vi "Multicore Simulator.vi"() -> ()   [LabVIEW 2016]
uses:
  Z:/LiSARD_Reference_Project/Multicore_1.6beta/CodeConverter/Controls/CommandLine.ctl
  Z:/LiSARD_Reference_Project/Multicore_1.6beta/CodeConverter/Controls/EX.Command.ctl
  Z:/LiSARD_Reference_Project/Multicore_1.6beta/CodeConverter/Controls/WB.Operation.ctl
  Z:/LiSARD_Reference_Project/Multicore_1.6beta/CodeConverter/SoftCoreCodeConverter.lvlib
panel:
  out "Output":dbl[](array[numeric])=[0.0, 1.0, 2.0, 3.0, 4.0, 5.0, 6.0, 7.0, 8.0, 9.0, 10.0, 11.0, 12.0, 13.0, 14.0, 15.0, 16.0, 17.0, 18.0, 19.0, 20.0, 21.0, 22.0, 23.0, 24.0, 25.0, 26.0, 27.0, 28.0, 29.0, 30.0, 0.0, 0.0, 0.0, 0.0, 0.0, 0.0, 0.0, 0.0, 0.0, 0.0, 0.0, 0.0, 0.0, 0.0, 0.0, 0.0, 0.0, 0.0, 0.0, 0.0, 0.0, 0.0, 0.0, 0.0, 0.0, 0.0, 0.0, 0.0, 0.0, 0.0, 0.0, 0.0, 0.0, 0.0, 0.0, 0.0, 0.0, 0.0, 0.0, 0.0, 0.0, 0.0, 0.0, 0.0, 0.0, 0.0, 0.0, 0.0, 0.0, 0.0, 0.0, 0.0, 0.0, 0.0, 0.0, 0.0, 0.0, 0.0, 0.0, 0.0, 0.0, 0.0, 0.0, 0.0, 0.0, 0.0, 0.0, 0.0, 0.0, 0.0, 0.0, 0.0, 0.0, 0.0, 0.0, 0.0, 0.0, 0.0, 0.0, 0.0, 0.0, 0.0, 0.0, 0.0, 0.0, 0.0, 0.0, 0.0, 0.0, 0.0, 0.0, 0.0, 0.0, 0.0, 0.0, 0.0, 0.0, 0.0, 0.0, 0.0, 0.0, 0.0, 0.0, 0.0, 0.0, 0.0, 0.0, 0.0, 0.0, 0.0, 0.0, 0.0, 0.0, 0.0, 0.0, 0.0, 0.0, 0.0, 0.0, 0.0, 0.0, 0.0, 0.0, 0.0, 0.0, 0.0, 0.0, 0.0, 0.0, 0.0, 0.0, 0.0, 0.0, 0.0, 0.0, 0.0, 0.0, 0.0, 0.0, 0.0, 0.0, 0.0, 0.0, 0.0, 0.0, 0.0, 0.0, 0.0, 0.0, 0.0, 0.0, 0.0, 0.0, 0.0, 0.0, 0.0, 0.0, 0.0, 0.0, 0.0, 0.0, 0.0, 0.0, 0.0, 0.0, 0.0, 0.0, 0.0, 0.0, 0.0, 0.0, 0.0, 0.0, 0.0, 0.0, 0.0, 0.0, 0.0, 0.0, 0.0, 0.0, 0.0, 0.0, 0.0, 0.0, 0.0, 0.0, 0.0, 0.0, 0.0, 0.0, 0.0, 0.0, 0.0, 0.0, 0.0, 0.0, 0.0, 0.0, 0.0, 0.0, 0.0, 0.0, 0.0, 0.0, 0.0, 0.0, 0.0, 0.0, 0.0, 0.0, 0.0, 0.0, 0.0, 0.0, 0.0, 0.0, 0.0, 0.0, 0.0, 0.0, 0.0, 0.0, 0.0]
  in  "CoreCode":T1[][](array[typedef])=[[{"Ex.Command"=enum."None", "Ex.AddressIn1"=1.0, "Ex.AddressIn2"=2.0, "WB.Command"=enum."Add", "WB.AddressOut"=3.0, "Bypass1"=0.0, "Bypass 2"=0.0}, {"Ex.Command"=enum."None", "Ex.AddressIn1"=9.0, "Ex.AddressIn2"=10.0, "WB.Command"=enum."Add", "WB.AddressOut"=11.0, "Bypass1"=0.0, "Bypass 2"=0.0}, {"Ex.Command"=enum."None", "Ex.AddressIn1"=23.0, "Ex.AddressIn2"=17.0, "WB.Command"=enum."Mul", "WB.AddressOut"=18.0, "Bypass1"=0.0, "Bypass 2"=0.0}, {"Ex.Command"=enum."None", "Ex.AddressIn1"=23.0, "Ex.AddressIn2"=23.0, "WB.Command"=enum."Mul", "WB.AddressOut"=24.0, "Bypass1"=0.0, "Bypass 2"=0.0}], [{"Ex.Command"=enum."None", "Ex.AddressIn1"=4.0, "Ex.AddressIn2"=5.0, "WB.Command"=enum."Mul", "WB.AddressOut"=6.0, "Bypass1"=0.0, "Bypass 2"=0.0}, {"Ex.Command"=enum."None", "Ex.AddressIn1"=11.0, "Ex.AddressIn2"=11.0, "WB.Command"=enum."Mul", "WB.AddressOut"=12.0, "Bypass1"=0.0, "Bypass 2"=0.0}, {"Ex.Command"=enum."None", "Ex.AddressIn1"=18.0, "Ex.AddressIn2"=18.0, "WB.Command"=enum."Mul", "WB.AddressOut"=19.0, "Bypass1"=0.0, "Bypass 2"=0.0}, {"Ex.Command"=enum."None", "Ex.AddressIn1"=23.0, "Ex.AddressIn2"=25.0, "WB.Command"=enum."Mul", "WB.AddressOut"=26.0, "Bypass1"=0.0, "Bypass 2"=0.0}], [{"Ex.Command"=enum."None", "Ex.AddressIn1"=3.0, "Ex.AddressIn2"=6.0, "WB.Command"=enum."Add", "WB.AddressOut"=7.0, "Bypass1"=0.0, "Bypass 2"=0.0}, {"Ex.Command"=enum."Sub", "Ex.AddressIn1"=13.0, "Ex.AddressIn2"=14.0, "WB.Command"=enum."Sub", "WB.AddressOut"=15.0, "Bypass1"=0.0, "Bypass 2"=0.0}, {"Ex.Command"=enum."None", "Ex.AddressIn1"=24.0, "Ex.AddressIn2"=20.0, "WB.Command"=enum."Add", "WB.AddressOut"=20.0, "Bypass1"=0.0, "Bypass 2"=0.0}, {"Ex.Command"=enum."Sub", "Ex.AddressIn1"=24.0, "Ex.AddressIn2"=26.0, "WB.Command"=enum."Sub", "WB.AddressOut"=27.0, "Bypass1"=0.0, "Bypass 2"=0.0}], [{"Ex.Command"=enum."None", "Ex.AddressIn1"=7.0, "Ex.AddressIn2"=8.0, "WB.Command"=enum."Mov", "WB.AddressOut"=1.0, "Bypass1"=3.0, "Bypass 2"=0.0}, {"Ex.Command"=enum."None", "Ex.AddressIn1"=15.0, "Ex.AddressIn2"=15.0, "WB.Command"=enum."Mul", "WB.AddressOut"=16.0, "Bypass1"=0.0, "Bypass 2"=0.0}, {"Ex.Command"=enum."None", "Ex.AddressIn1"=19.0, "Ex.AddressIn2"=20.0, "WB.Command"=enum."Add", "WB.AddressOut"=22.0, "Bypass1"=0.0, "Bypass 2"=0.0}, {"Ex.Command"=enum."None", "Ex.AddressIn1"=25.0, "Ex.AddressIn2"=25.0, "WB.Command"=enum."Mul", "WB.AddressOut"=28.0, "Bypass1"=0.0, "Bypass 2"=0.0}], [{"Ex.Command"=enum."Sub", "Ex.AddressIn1"=1.0, "Ex.AddressIn2"=4.0, "WB.Command"=enum."Sub", "WB.AddressOut"=2.0, "Bypass1"=0.0, "Bypass 2"=0.0}, {"Ex.Command"=enum."Sub", "Ex.AddressIn1"=12.0, "Ex.AddressIn2"=16.0, "WB.Command"=enum."Sub", "WB.AddressOut"=10.0, "Bypass1"=0.0, "Bypass 2"=0.0}, {"Ex.Command"=enum."None", "Ex.AddressIn1"=22.0, "Ex.AddressIn2"=23.0, "WB.Command"=enum."Mov", "WB.AddressOut"=21.0, "Bypass1"=0.0, "Bypass 2"=0.0}, {"Ex.Command"=enum."None", "Ex.AddressIn1"=27.0, "Ex.AddressIn2"=28.0, "WB.Command"=enum."Add", "WB.AddressOut"=29.0, "Bypass1"=0.0, "Bypass 2"=0.0}]]
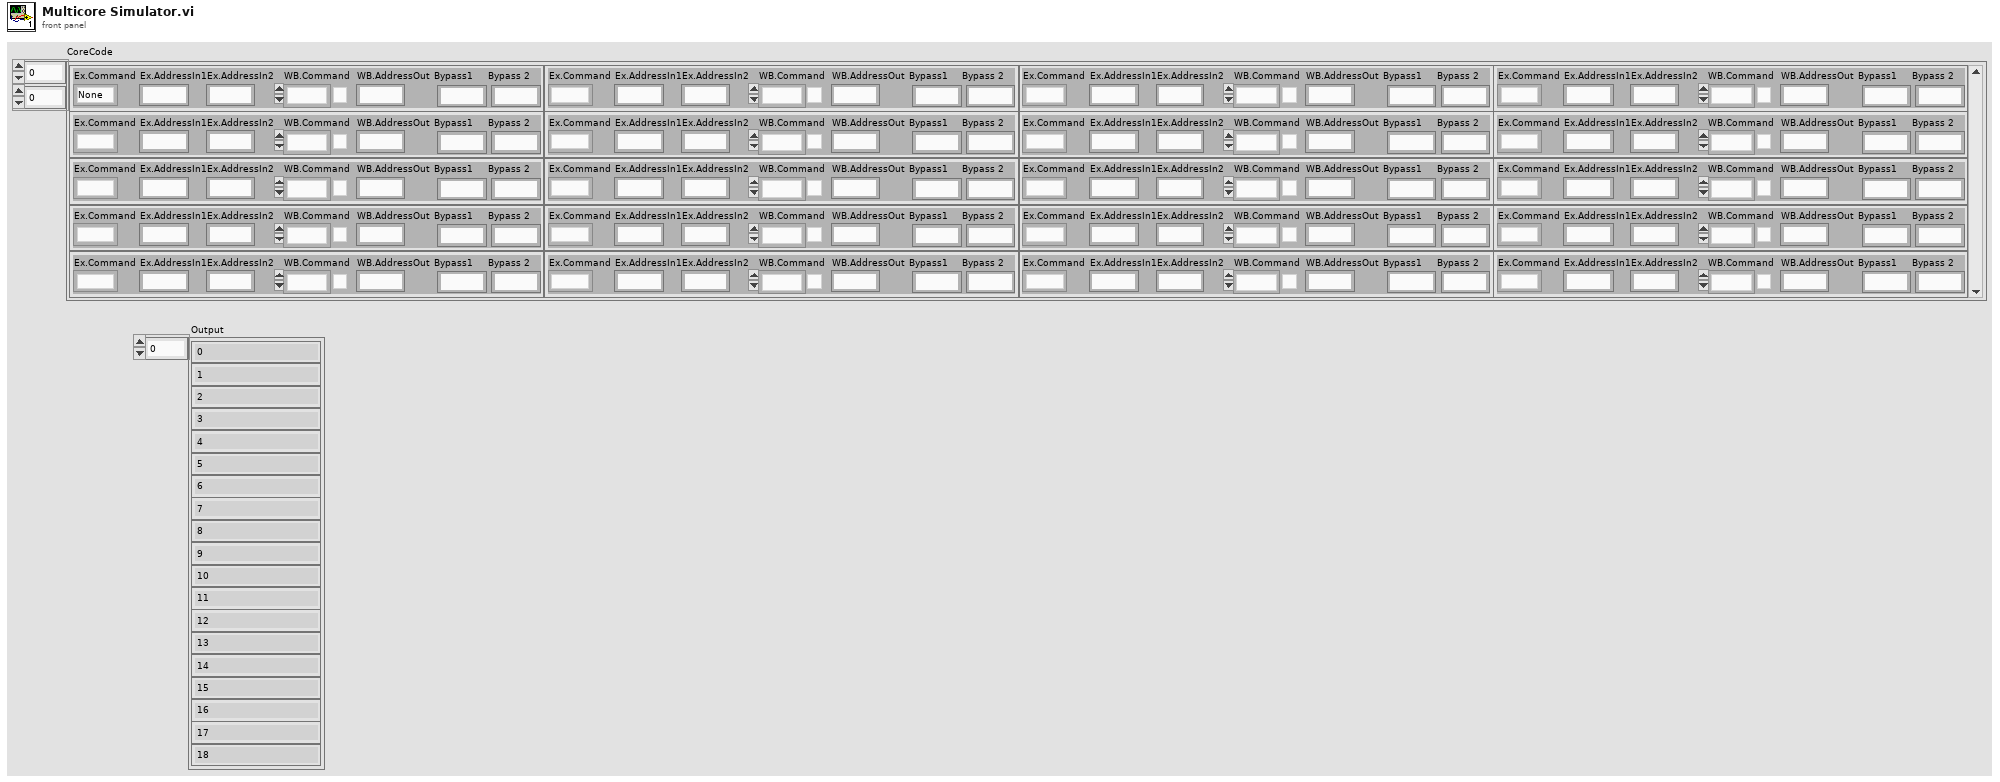
[diagram p1: front panel]
types:
  T1 = typedef "SoftCoreCodeConverter.lvlib/CommandLine.ctl" = cluster{"Ex.Command":T2, "Ex.AddressIn1":fxp<+,16,16>, "Ex.AddressIn2":fxp<+,16,16>, "WB.Command":T3, "WB.AddressOut":fxp<+,16,16>, "Bypass1":fxp<+,2,2>, "Bypass 2":fxp<+,2,2>}
  T2 = typedef "SoftCoreCodeConverter.lvlib/EX.Command.ctl" = enum8{"Default", "Sub", "None", "Fuse", "Abs", "AbsSub", "Const"}
  T3 = typedef "SoftCoreCodeConverter.lvlib/WB.Operation.ctl" = enum8{"In", "Out", "Mov", "Add", "Sub", "Mul", "Div", "None", "Sqr", "Sin", "Cos", "Sgl2Dbl", "Dbl2Int", "Int2Dbl", "Mlookup", "Dbl2Sgl", "G_IsPOS", "G_IsNEG", "G_IsNULL", "G_IsNNULL", "G_IsNAN", "G_IsNNAN", "G_IsIFTY", "G_IsNIFTY", "reserved_0", "reserved_1", "reserved_2", "reserved_3", "reserved_4", "reserved_5", "reserved_6", "reserved_7"}
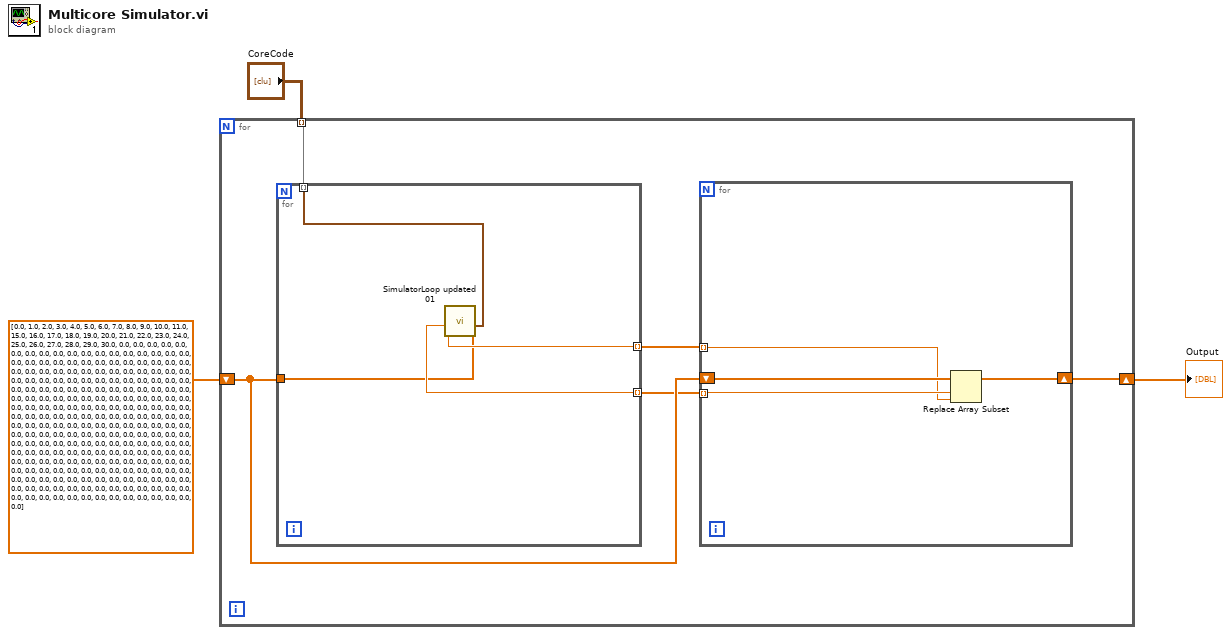
[diagram p0: block diagram]
diagram:
  n1 = for {
    shift-right: [w7] -> w2
    shift-left: dbl[] [0.0, 1.0, 2.0, 3.0, 4.0, 5.0, 6.0, 7.0, 8.0, 9.0, 10.0, 11.0, 15.0, 16.0, 17.0, 18.0, 19.0, 20.0, 21.0, 22.0, 23.0, 24.0, 25.0, 26.0, 27.0, 28.0, 29.0, 30.0, 0.0, 0.0, 0.0, 0.0, 0.0, 0.0, 0.0, 0.0, 0.0, 0.0, 0.0, 0.0, 0.0, 0.0, 0.0, 0.0, 0.0, 0.0, 0.0, 0.0, 0.0, 0.0, 0.0, 0.0, 0.0, 0.0, 0.0, 0.0, 0.0, 0.0, 0.0, 0.0, 0.0, 0.0, 0.0, 0.0, 0.0, 0.0, 0.0, 0.0, 0.0, 0.0, 0.0, 0.0, 0.0, 0.0, 0.0, 0.0, 0.0, 0.0, 0.0, 0.0, 0.0, 0.0, 0.0, 0.0, 0.0, 0.0, 0.0, 0.0, 0.0, 0.0, 0.0, 0.0, 0.0, 0.0, 0.0, 0.0, 0.0, 0.0, 0.0, 0.0, 0.0, 0.0, 0.0, 0.0, 0.0, 0.0, 0.0, 0.0, 0.0, 0.0, 0.0, 0.0, 0.0, 0.0, 0.0, 0.0, 0.0, 0.0, 0.0, 0.0, 0.0, 0.0, 0.0, 0.0, 0.0, 0.0, 0.0, 0.0, 0.0, 0.0, 0.0, 0.0, 0.0, 0.0, 0.0, 0.0, 0.0, 0.0, 0.0, 0.0, 0.0, 0.0, 0.0, 0.0, 0.0, 0.0, 0.0, 0.0, 0.0, 0.0, 0.0, 0.0, 0.0, 0.0, 0.0, 0.0, 0.0, 0.0, 0.0, 0.0, 0.0, 0.0, 0.0, 0.0, 0.0, 0.0, 0.0, 0.0, 0.0, 0.0, 0.0, 0.0, 0.0, 0.0, 0.0, 0.0, 0.0, 0.0, 0.0, 0.0, 0.0, 0.0, 0.0, 0.0, 0.0, 0.0, 0.0, 0.0, 0.0, 0.0, 0.0, 0.0, 0.0, 0.0, 0.0, 0.0, 0.0, 0.0, 0.0, 0.0, 0.0, 0.0, 0.0, 0.0, 0.0, 0.0, 0.0, 0.0, 0.0, 0.0, 0.0, 0.0, 0.0, 0.0, 0.0, 0.0, 0.0, 0.0, 0.0, 0.0, 0.0, 0.0, 0.0, 0.0, 0.0, 0.0, 0.0, 0.0, 0.0, 0.0, 0.0, 0.0, 0.0, 0.0, 0.0, 0.0, 0.0, 0.0, 0.0, 0.0, 0.0, 0.0, 0.0, 0.0, 0.0, 0.0, 0.0, 0.0, 0.0, 0.0, 0.0, 0.0, 0.0, 0.0, 0.0] ("DataMemory/Fxp") -> [w8]
    tunnel: "CoreCode" -> [w6] mode=indexing
    n2 = for {
      tunnel: w8 -> [w13]
      tunnel: w6 -> [w16] mode=indexing
      tunnel: [w15] -> w5 mode=indexing
      tunnel: [w14] -> w4 mode=indexing
      n3 = call "SimulatorLoop updated 01.vi"("DataMemory/Fxp"=w13, "CodeLine"=w16) -> ("Data"=w15:dbl, "Address"=w14:dbl)  [unwired: 8 in]
    }
    n4 = for {
      shift-right: [w12] -> w7
      shift-left: w8 -> [w11]
      tunnel: w5 -> [w9] mode=indexing
      tunnel: w4 -> [w10] mode=indexing
      n5 = Replace Array Subset(array=w11, new element=w9, index=w10) -> (w12:dbl[])
    }
  }
  "Output" <- w2
